vi "ShapeOKCons.vi"() -> ()   [LabVIEW 2014]
doc: "This example performs a serial port write and a serial port read. The parameters set for the serial port must match the parameters of the connected instrument or device. The VISA Configure Serial Port VI sets the configuration parameters. The front panel displays the controls used to configure the basic parameters, such as baud rate, data bits, and parity. The VI passes the VISA resource name to other VIs that perform operations on that VISA resource. The VISA Write function sends a command to the serial device and the VISA Read function returns data based on the command. The VISA Close function then closes the reference to the serial device. It is important to close the reference; otherwise, further communication through that port might not be possible."
uses:
  School/MultiSim/LabVIEW 2014/examples/Instrument IO/Serial/support/Serial - Settings.ctl
  HeadControl.ctl
  <vilib>/Instr/_visa.llb/VISA Configure Serial Port (Instr).vi
panel:
  in  "Read File":bool
  in  "stop":bool
  in  "Enqueue Element":bool
  in  "Command":string="*IDN?\n"
  in  "MoveHead":T1
  out "HeadPosition":cluster{"X":i16, "Y":i16, "Z":i16}
  out "error out":errorcluster
  out "Response":string
  out "Serial Settings:Number of Bytes at Serial Port":u32
  in  "Serial Settings":T2={"baud rate"=9600, "data bits"=8, "parity"=enum."None", "stop bits"=10, "flow control"=0} {"flow control" items=["None"=0, "XON/XOFF"=1, "RTS/CTS"=2, "DTR/DSR"=4]; "stop bits" items=["1.0"=10, "1.5"=15, "2.0"=20]; "data bits" min=5 max=8 step=1; "baud rate" items=["75"=75, "110"=110, "134"=134, "150"=150, "300"=300, "600"=600, "1200"=1200, "1800"=1800, "2400"=2400, "4800"=4800, "7200"=7200, "9600"=9600, "14400"=14400, "19200"=19200, "28800"=28800, "38400"=38400, "56000"=56000, "57600"=57600, "115200"=115200, "128000"=128000, "230400"=230400]}
  in  "VISA resource name":refnum<visa-resource-name>="COM1"
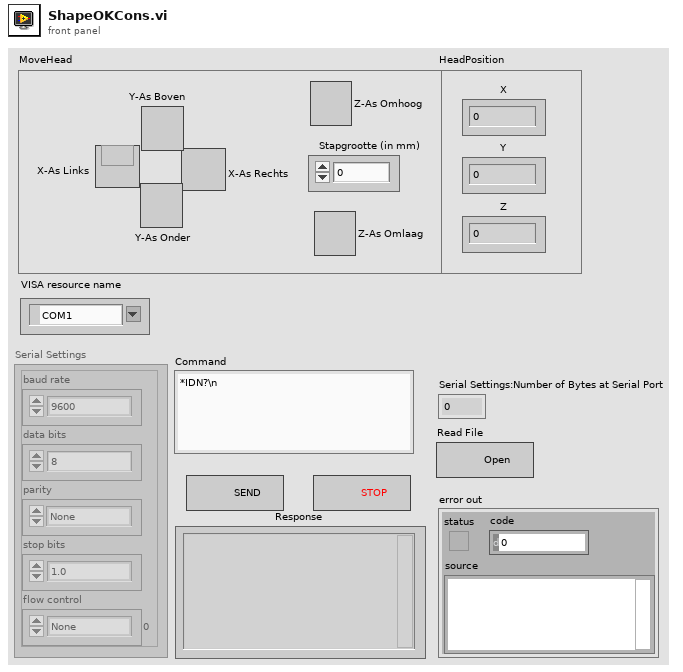
[diagram p1: front panel]
types:
  T1 = typedef "HeadControl.ctl" = cluster{"X-As Links":bool, "X-As Rechts":bool, "Y-As Boven":bool, "Y-As Onder":bool, "Z-As Omhoog":bool, "Z-As Omlaag":bool, "Stapgrootte (in mm)":i8}
  T2 = typedef "Serial - Settings.ctl" = cluster{"baud rate":u32, "data bits":u16, "parity":enum16{"None", "Odd", "Even", "Mark", "Space"}, "stop bits":u16, "flow control":u16}
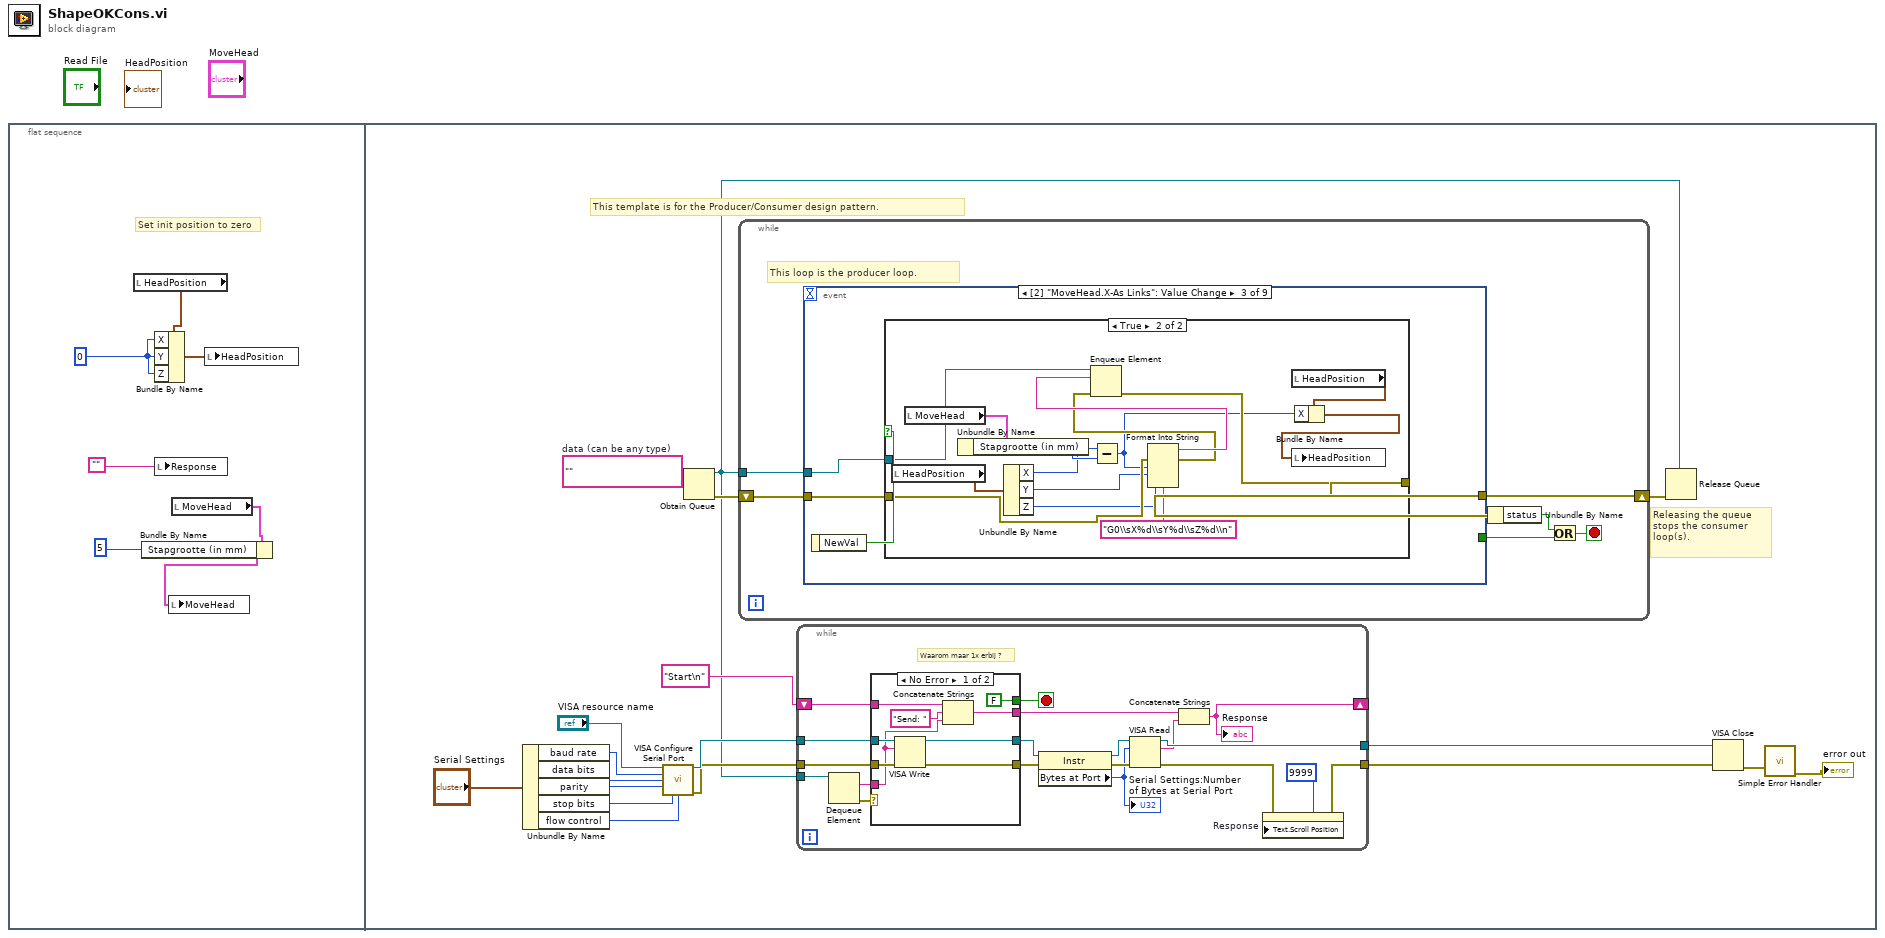
[diagram p0: block diagram]
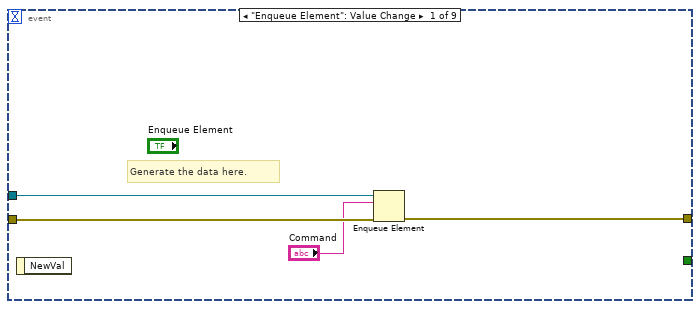
[diagram p2: hidden frame]
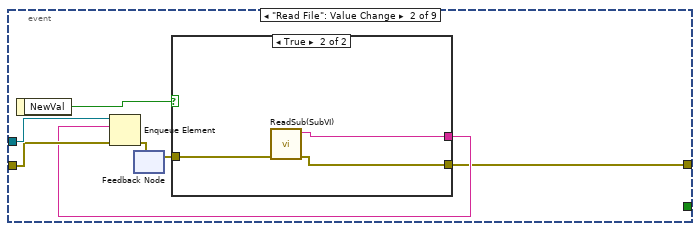
[diagram p3: hidden frame]
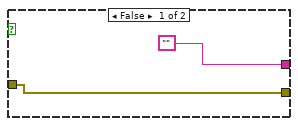
[diagram p4: hidden frame]
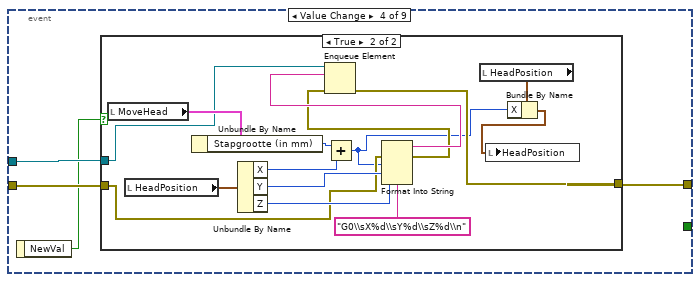
[diagram p6: hidden frame]
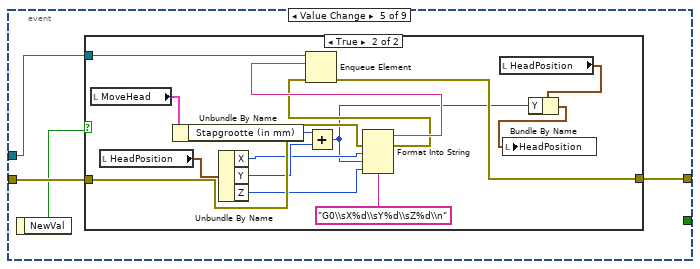
[diagram p8: hidden frame]
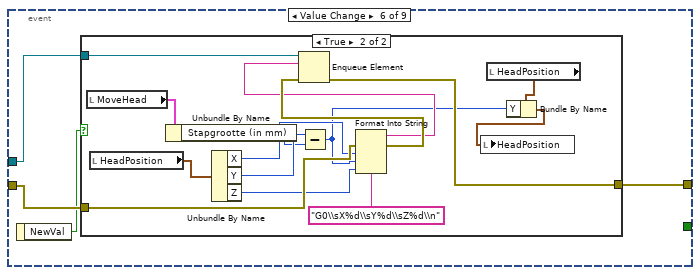
[diagram p10: hidden frame]
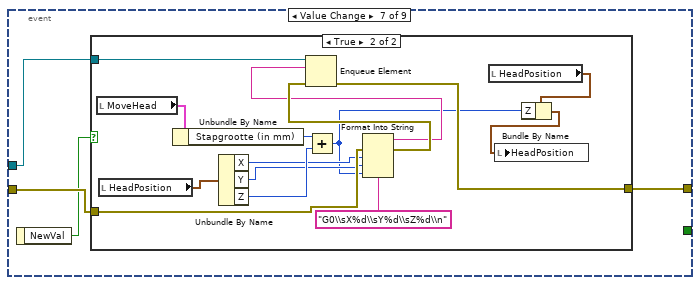
[diagram p12: hidden frame]
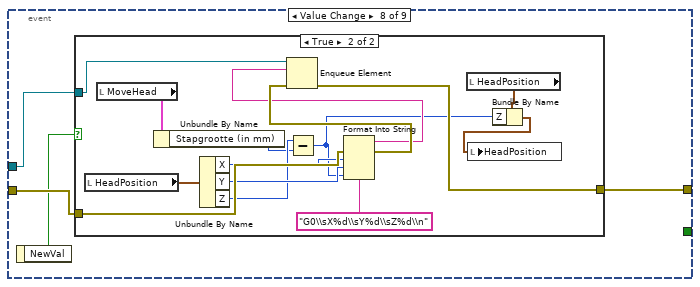
[diagram p14: hidden frame]
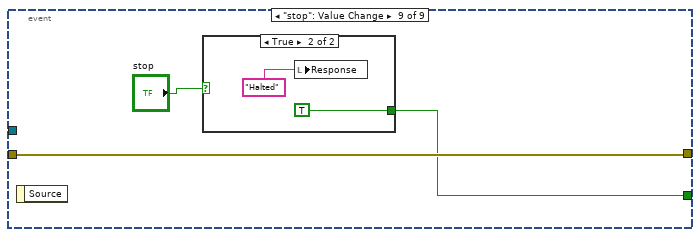
[diagram p16: hidden frame]
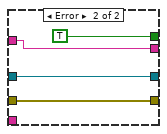
[diagram p18: hidden frame]
diagram:
  n1 = flat-sequence {
    frame #0 {
      w5 = 0
      # "Set init position to zero"
      n2 = local read "HeadPosition"() -> (w6:cluster{"X":i16, "Y":i16, "Z":i16})
      n3 = Bundle By Name(cluster=w6, "X"=w5, "Y"=w5, "Z"=w5) -> (w7:cluster{"X":i16, "Y":i16, "Z":i16})
      n4 = local write "Response"("") -> ()
      n5 = local read "MoveHead"() -> (w3:T1)
      n6 = Bundle By Name(cluster=w3, "Stapgrootte (in mm)"=5) -> (w1:T1)
      n7 = local write "MoveHead"(w1) -> ()
      n8 = local write "HeadPosition"(w7) -> ()
    }
    frame #1 {
      w10 = ""  # data (can be any type)
      # "Releasing the queue stops the consumer loop(s)."
      # "This template is for the Producer/Consumer design pattern."
      n9 = Unbundle By Name("Serial Settings") -> ("baud rate"=w23:u32, "data bits"=w22:u16, "parity"=w21:enum16{"None", "Odd", "Even", "Mark", "Space"}, "stop bits"=w20:u16, "flow control"=w19:u16)
      n10 = call-poly "VISA Configure Serial Port"("VISA resource name"="VISA resource name", "baud rate (9600)"=w23, "data bits (8)"=w22, "parity (0:none)"=w21, "stop bits (10: 1 bit)"=w20, "flow control (0:none)"=w19) -> ("VISA resource name out"=w15:refnum<visa-resource-name>, "error out"=w14:errorcluster)  [unwired: 3 in, 5 out]
      n11 = Obtain Queue(element data type=w10) -> (queue out=w9:refnum<queue>, error out=w12:errorcluster)  [unwired: 4 in, 1 out]
      n12 = while {
        shift-right: [w27] -> w11
        shift-left: w12 -> [w30]
        tunnel: w9 -> [w31]
        stop <- w28 stop-if-true
        # "This loop is the producer loop."
        n13 = event shown="[2] \"MoveHead.X-As Links\": Value Change" {
          selector: _ -> [_ _ _ _ _ _ _ _ _]
          dyn-events: _ -> [_ _ _ _ _ _ _ _ _]
          timeout: _ -> [_ _ _ _ _ _ _ _ _]
          tunnel: w31 -> [w35 w41 w51 w71 w91 w111 w131 w151 _]
          tunnel: w30 -> [w34 w40 w49 w70 w89 w110 w130 w150 w170]
          tunnel: [w33 w38 w50 w69 w90 w108 w128 w148 w170] -> w27
          tunnel: [_ _ _ _ _ _ _ _ w168] -> w29
          event "Enqueue Element": Value Change {
            # "Generate the data here."
            n14 = event-data() -> ()  [unwired: 1 in, 1 out]
            n15 = Enqueue Element(queue=w35, element="Command", error in (no error)=w34) -> (error out=w33:errorcluster)  [unwired: 1 in, 2 out]
          }
          event "Read File": Value Change {
            n16 = event-data() -> ("NewVal"=w42:bool)  [unwired: 1 in]
            n17 = feedback #1() -> (w36:errorcluster)  [unwired: 1 in]
            n18 = case shown="True" w42 {
              tunnel: ["" w47] -> w39
              tunnel: w36 -> [w43 w46]
              tunnel: [w43 w45] -> w38
              frame False {
              }
              frame True {
                n19 = call "ReadSub(SubVI).vi"("error in"=w46) -> ("error out"=w45:errorcluster, "Output"=w47:string)  [unwired: 9 in]
              }
            }
            n20 = Enqueue Element(queue=w41, element=w39, error in (no error)=w40) -> (error out=w37:errorcluster)  [unwired: 1 in, 2 out]
            n21 = feedback-in #1(w37) -> ()
          }
          event Value Change {
            n22 = event-data() -> ("NewVal"=w48:bool)  [unwired: 1 in]
            n23 = case shown="True" w48 {
              tunnel: w51 -> [_ w64]
              tunnel: [w52 w62] -> w50
              tunnel: w49 -> [w52 w60]
              frame False {
              }
              frame True {
                n24 = local read "HeadPosition"() -> (w66:cluster{"X":i16, "Y":i16, "Z":i16})
                n25 = local read "MoveHead"() -> (w67:T1)
                n26 = Unbundle By Name(w67) -> ("Stapgrootte (in mm)"=w54:i8)
                n27 = Unbundle By Name(w66) -> ("X"=w53:i16, "Y"=w58:i16, "Z"=w59:i16)
                n28 = Subtract(x=w53, y=w54) -> (x-y=w57:i16)
                n29 = Format Into String(format string="G0\\sX%d\\sY%d\\sZ%d\\n", error in=w60, w57, w58, w59) -> (resulting string=w63:string, error out=w61:errorcluster)  [unwired: 1 in]
                n30 = Enqueue Element(queue=w64, element=w63, error in (no error)=w61) -> (error out=w62:errorcluster)  [unwired: 1 in, 2 out]
                n31 = local read "HeadPosition"() -> (w56:cluster{"X":i16, "Y":i16, "Z":i16})
                n32 = Bundle By Name(cluster=w56, "X"=w57) -> (w55:cluster{"X":i16, "Y":i16, "Z":i16})
                n33 = local write "HeadPosition"(w55) -> ()
              }
            }
          }
          event Value Change {
            n34 = event-data() -> ("NewVal"=w68:bool)  [unwired: 1 in]
            n35 = case shown="True" w68 {
              tunnel: w71 -> [_ w78]
              tunnel: w70 -> [w72 w77]
              tunnel: [w72 w76] -> w69
              frame False {
              }
              frame True {
                n36 = local read "MoveHead"() -> (w80:T1)
                n37 = local read "HeadPosition"() -> (w79:cluster{"X":i16, "Y":i16, "Z":i16})
                n38 = Unbundle By Name(w80) -> ("Stapgrootte (in mm)"=w86:i8)
                n39 = Unbundle By Name(w79) -> ("X"=w87:i16, "Y"=w84:i16, "Z"=w83:i16)
                n40 = Add(x=w86, y=w87) -> (x+y=w73:i16)
                n41 = Format Into String(format string="G0\\sX%d\\sY%d\\sZ%d\\n", error in=w77, w73, w84, w83) -> (resulting string=w82:string, error out=w81:errorcluster)  [unwired: 1 in]
                n42 = Enqueue Element(queue=w78, element=w82, error in (no error)=w81) -> (error out=w76:errorcluster)  [unwired: 1 in, 2 out]
                n43 = local read "HeadPosition"() -> (w75:cluster{"X":i16, "Y":i16, "Z":i16})
                n44 = Bundle By Name(cluster=w75, "X"=w73) -> (w74:cluster{"X":i16, "Y":i16, "Z":i16})
                n45 = local write "HeadPosition"(w74) -> ()
              }
            }
          }
          event Value Change {
            n46 = event-data() -> ("NewVal"=w88:bool)  [unwired: 1 in]
            n47 = case shown="True" w88 {
              tunnel: w91 -> [_ w104]
              tunnel: [w92 w103] -> w90
              tunnel: w89 -> [w92 w102]
              frame False {
              }
              frame True {
                n48 = local read "MoveHead"() -> (w101:T1)
                n49 = local read "HeadPosition"() -> (w99:cluster{"X":i16, "Y":i16, "Z":i16})
                n50 = Unbundle By Name(w101) -> ("Stapgrootte (in mm)"=w100:i8)
                n51 = Unbundle By Name(w99) -> ("X"=w97:i16, "Y"=w98:i16, "Z"=w96:i16)
                n52 = Add(x=w100, y=w98) -> (x+y=w93:i16)
                n53 = Format Into String(format string="G0\\sX%d\\sY%d\\sZ%d\\n", error in=w102, w97, w93, w96) -> (resulting string=w106:string, error out=w105:errorcluster)  [unwired: 1 in]
                n54 = Enqueue Element(queue=w104, element=w106, error in (no error)=w105) -> (error out=w103:errorcluster)  [unwired: 1 in, 2 out]
                n55 = local read "HeadPosition"() -> (w95:cluster{"X":i16, "Y":i16, "Z":i16})
                n56 = Bundle By Name(cluster=w95, "Y"=w93) -> (w94:cluster{"X":i16, "Y":i16, "Z":i16})
                n57 = local write "HeadPosition"(w94) -> ()
              }
            }
          }
          event Value Change {
            n58 = event-data() -> ("NewVal"=w109:bool)  [unwired: 1 in]
            n59 = case shown="True" w109 {
              tunnel: w111 -> [_ w122]
              tunnel: w110 -> [w112 w121]
              tunnel: [w112 w120] -> w108
              frame False {
              }
              frame True {
                n60 = local read "MoveHead"() -> (w123:T1)
                n61 = local read "HeadPosition"() -> (w124:cluster{"X":i16, "Y":i16, "Z":i16})
                n62 = Unbundle By Name(w123) -> ("Stapgrootte (in mm)"=w113:i8)
                n63 = Unbundle By Name(w124) -> ("X"=w119:i16, "Y"=w114:i16, "Z"=w118:i16)
                n64 = Subtract(x=w114, y=w113) -> (x-y=w115:i16)
                n65 = Format Into String(format string="G0\\sX%d\\sY%d\\sZ%d\\n", error in=w121, w119, w115, w118) -> (resulting string=w126:string, error out=w127:errorcluster)  [unwired: 1 in]
                n66 = Enqueue Element(queue=w122, element=w126, error in (no error)=w127) -> (error out=w120:errorcluster)  [unwired: 1 in, 2 out]
                n67 = local read "HeadPosition"() -> (w117:cluster{"X":i16, "Y":i16, "Z":i16})
                n68 = Bundle By Name(cluster=w117, "Y"=w115) -> (w116:cluster{"X":i16, "Y":i16, "Z":i16})
                n69 = local write "HeadPosition"(w116) -> ()
              }
            }
          }
          event Value Change {
            n70 = event-data() -> ("NewVal"=w129:bool)  [unwired: 1 in]
            n71 = case shown="True" w129 {
              tunnel: w131 -> [_ w141]
              tunnel: w130 -> [w132 w140]
              tunnel: [w132 w139] -> w128
              frame False {
              }
              frame True {
                n72 = local read "MoveHead"() -> (w143:T1)
                n73 = local read "HeadPosition"() -> (w144:cluster{"X":i16, "Y":i16, "Z":i16})
                n74 = Unbundle By Name(w143) -> ("Stapgrootte (in mm)"=w142:i8)
                n75 = Unbundle By Name(w144) -> ("X"=w137:i16, "Y"=w136:i16, "Z"=w138:i16)
                n76 = Add(x=w142, y=w138) -> (x+y=w133:i16)
                n77 = Format Into String(format string="G0\\sX%d\\sY%d\\sZ%d\\n", error in=w140, w137, w136, w133) -> (resulting string=w146:string, error out=w147:errorcluster)  [unwired: 1 in]
                n78 = Enqueue Element(queue=w141, element=w146, error in (no error)=w147) -> (error out=w139:errorcluster)  [unwired: 1 in, 2 out]
                n79 = local read "HeadPosition"() -> (w135:cluster{"X":i16, "Y":i16, "Z":i16})
                n80 = Bundle By Name(cluster=w135, "Z"=w133) -> (w134:cluster{"X":i16, "Y":i16, "Z":i16})
                n81 = local write "HeadPosition"(w134) -> ()
              }
            }
          }
          event Value Change {
            n82 = event-data() -> ("NewVal"=w149:bool)  [unwired: 1 in]
            n83 = case shown="True" w149 {
              tunnel: w151 -> [_ w162]
              tunnel: w150 -> [w152 w161]
              tunnel: [w152 w160] -> w148
              frame False {
              }
              frame True {
                n84 = local read "HeadPosition"() -> (w163:cluster{"X":i16, "Y":i16, "Z":i16})
                n85 = local read "MoveHead"() -> (w164:T1)
                n86 = Unbundle By Name(w164) -> ("Stapgrootte (in mm)"=w153:i8)
                n87 = Unbundle By Name(w163) -> ("X"=w159:i16, "Y"=w158:i16, "Z"=w154:i16)
                n88 = Subtract(x=w154, y=w153) -> (x-y=w155:i16)
                n89 = Format Into String(format string="G0\\sX%d\\sY%d\\sZ%d\\n", error in=w161, w159, w158, w155) -> (resulting string=w166:string, error out=w167:errorcluster)  [unwired: 1 in]
                n90 = Enqueue Element(queue=w162, element=w166, error in (no error)=w167) -> (error out=w160:errorcluster)  [unwired: 1 in, 2 out]
                n91 = local read "HeadPosition"() -> (w157:cluster{"X":i16, "Y":i16, "Z":i16})
                n92 = Bundle By Name(cluster=w157, "Z"=w155) -> (w156:cluster{"X":i16, "Y":i16, "Z":i16})
                n93 = local write "HeadPosition"(w156) -> ()
              }
            }
          }
          event "stop": Value Change {
            n94 = event-data() -> ()  [unwired: 1 in, 1 out]
            n95 = case shown="True" "stop" {
              selector: "stop" -> [w171 _]
              tunnel: [w171 TRUE] -> w168
              frame False {
              }
              frame True {
                n96 = local write "Response"("Halted") -> ()
              }
            }
          }
        }
        n97 = Unbundle By Name(w27) -> ("status"=w26:bool)
        n98 = Or(x=w26, y=w29) -> (x .or. y?=w28:bool)
      }
      n99 = while {
        tunnel: w15 -> [w191]
        tunnel: w14 -> [w190]
        tunnel: [w192] -> w8
        tunnel: [w174] -> w18
        shift-right: [w183] -> _
        shift-left: "Start\n" -> [w182]
        tunnel: w9 -> [w180]
        stop <- w177 stop-if-true
        # "Waarom maar 1x erbij ?"
        n100 = Dequeue Element(queue=w180) -> (element=w178:string, error out=w179:errorcluster)  [unwired: 2 in, 2 out]
        n101 = case shown="No Error" w179 {
          tunnel: w191 -> [w201 w205]
          tunnel: w190 -> [w200 w204]
          tunnel: [w198 w205] -> w185
          tunnel: [w199 w204] -> w189
          tunnel: w182 -> [w196 w203]
          tunnel: [w195 w203] -> w181
          tunnel: w178 -> [w193 _]
          tunnel: [FALSE TRUE] -> w177
          frame No Error {
            n102 = VISA Write(VISA resource name=w201, write buffer=w193, error in (no error)=w200) -> (VISA resource name out=w198:refnum<visa-resource-name>, error out=w199:errorcluster)  [unwired: 1 out]
            n103 = Concatenate Strings(w196, "Send: ", w193) -> (w195:string)
          }
          frame Error {
          }
        }
        n104 = property class="Instr"(reference=w185, error in=w189) -> (reference out=w188:refnum<visa-resource-name>, error out=w187:errorcluster, "Bytes at Port"=w186:u32)
        "Serial Settings:Number of Bytes at Serial Port" <- w186
        n105 = VISA Read(VISA resource name=w188, byte count=w186, error in (no error)=w187) -> (VISA resource name out=w192:refnum<visa-resource-name>, read buffer=w184:string, error out=w175:errorcluster)  [unwired: 1 out]
        n106 = Concatenate Strings(w181, w184) -> (w183:string)
        "Response" <- w183
        n107 = property on="Response" class="Str"(error in=w175, "Text.Scroll Position"=u32 9999) -> (error out=w174:errorcluster)  [unwired: 1 in, 1 out]
      }
      n108 = Release Queue(queue=w9, error in (no error)=w11) -> ()  [unwired: 1 in, 3 out]
      n109 = VISA Close(VISA resource name=w8, error in (no error)=w18) -> (error out=w17:errorcluster)
      n110 = call <vilib>:"Simple Error Handler.vi"("error in (no error)"=w17) -> ("error out"=→"error out":errorcluster)  [unwired: 4 in, 4 out]
    }
  }
